vi "polygon_angle.vi"(0 "polygon":dbl[][](array[numeric])) -> (1 "kx":dbl, 2 "ky":dbl, 3 "z-angle":dbl)   [LabVIEW 2011]
panel:
  # "x1 y1 z1\nx2 y2 z2\nx3 y3 z3"
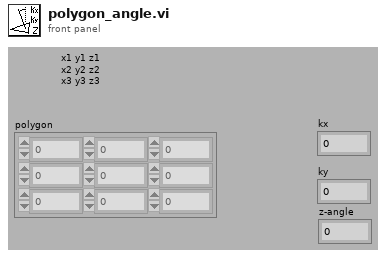
[diagram p1: front panel]
types:
  T1 = cluster{"AxB[0]":dbl, "AxB[1]":dbl, "AxB[2]":dbl}
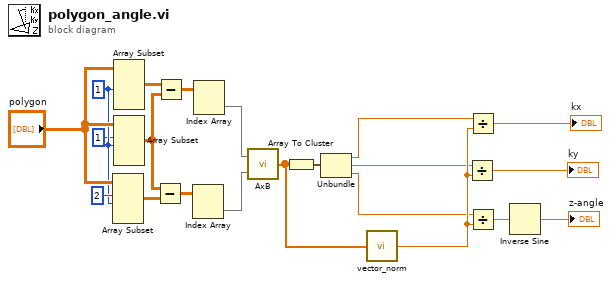
[diagram p0: block diagram]
diagram:
  w12 = 1 ("length")
  n1 = Array Subset(array="polygon", index (row)=2 ("index"), length (row)=w12) -> (w16:dbl[][])  [unwired: 2 in]
  n2 = Array Subset(array="polygon", length (row)=w12) -> (w14:dbl[][])  [unwired: 3 in]
  n3 = Array Subset(array="polygon", index (row)=1 ("index"), length (row)=w12) -> (w15:dbl[][])  [unwired: 2 in]
  n4 = Subtract(x=w15, y=w16) -> (x-y=w19:dbl[][])
  n5 = Subtract(x=w14, y=w15) -> (x-y=w17:dbl[][])
  n6 = Index Array(array=w19) -> (element=w20:dbl[])  [unwired: 2 in]
  n7 = Index Array(array=w17) -> (element=w18:dbl[])  [unwired: 2 in]
  n8 = call "AxB.vi"("B"=w20, "A"=w18) -> ("AxB"=w3:dbl[])
  n9 = Array To Cluster(array=w3) -> (cluster=w7:T1)
  n10 = Unbundle(w7) -> ("AxB[0]"=w6:dbl, "AxB[1]"=w5:dbl, "AxB[2]"=w4:dbl)
  n11 = call "vector_norm.vi"("A"=w3) -> ("norm"=w10:dbl)
  n12 = Divide(x=w5, y=w10) -> (x/y=→"ky":dbl)
  n13 = Divide(x=w6, y=w10) -> (x/y=→"kx":dbl)
  n14 = Divide(x=w4, y=w10) -> (x/y=w9:dbl)
  n15 = Inverse Sine(1:w9) -> (0:→"z-angle":dbl)
